vi "Distance.vi"(0 "X1":dbl, 1 "Y1":dbl, 2 "X2":dbl, 3 "Y2":dbl, 4 "X3":dbl, 5 "Y3":dbl, 6 "x4":dbl, 8 "Y":dbl, 9 "Y4":dbl, 10 "X":dbl) -> (14 "a2":dbl, 16 "a1":dbl, 17 "a3":dbl, 18 "Ra1":dbl, 19 "a4":dbl, 20 "A1":dbl, 21 "Ra2":dbl, 22 "Ra3":dbl, 23 "A2":dbl, 24 "Ra4":dbl, 25 "A3":dbl, 26 "A4":dbl)   [LabVIEW 2012]
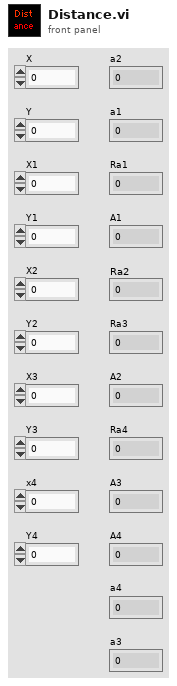
[diagram p1: front panel]
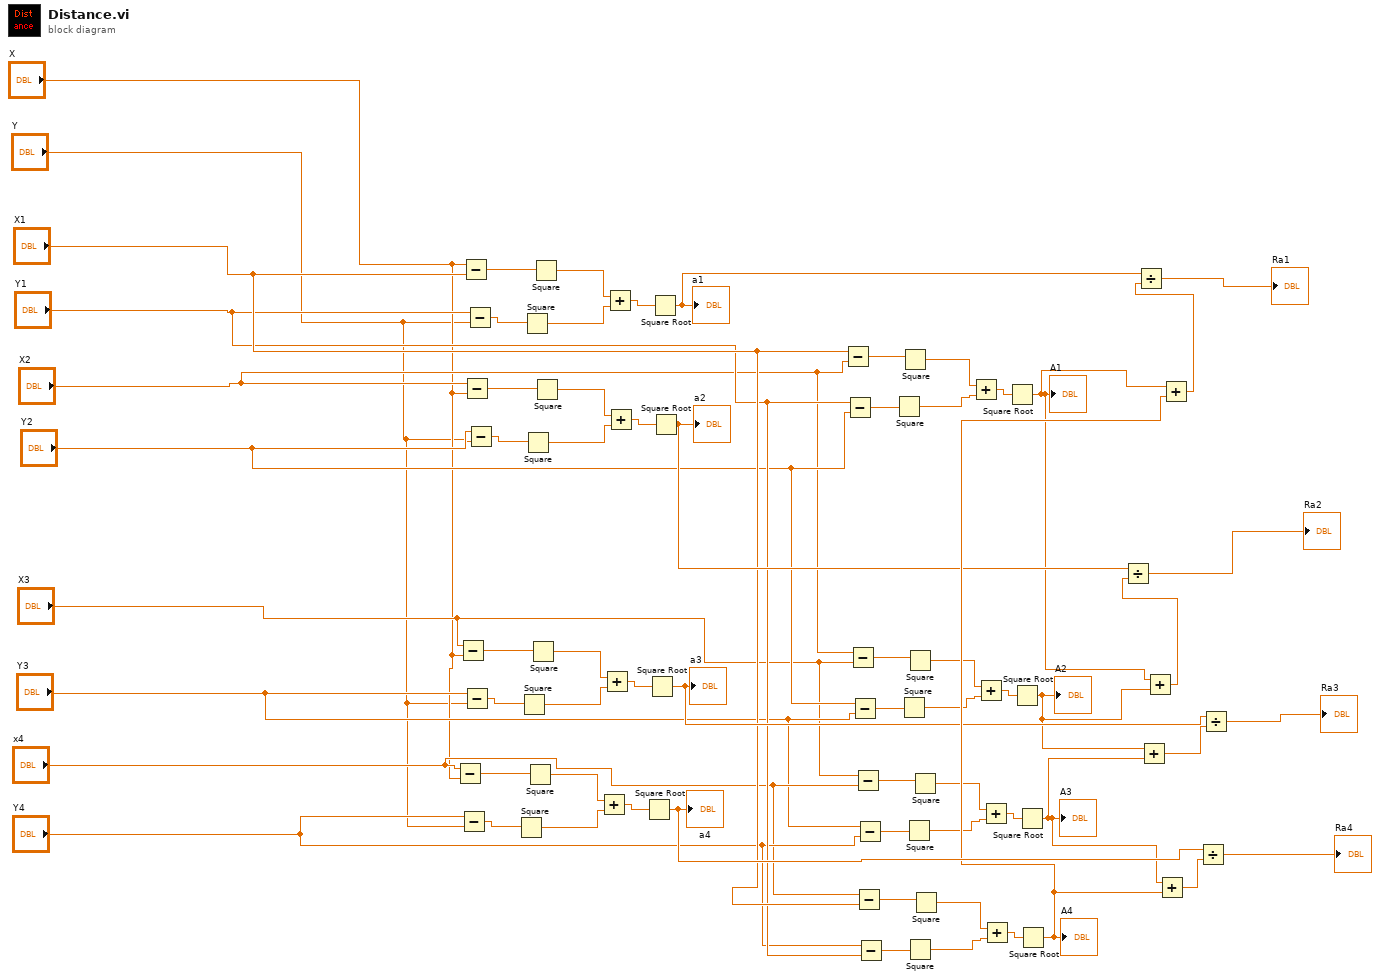
[diagram p0: block diagram]
diagram:
  n1 = Subtract(x="x4", y="X") -> (x-y=w17:dbl)
  n2 = Subtract(x="X3", y="X") -> (x-y=w12:dbl)
  n3 = Subtract(x="Y4", y="Y") -> (x-y=w18:dbl)
  n4 = Subtract(x="X", y="X1") -> (x-y=w2:dbl)
  n5 = Subtract(x="X2", y="X") -> (x-y=w7:dbl)
  n6 = Subtract(x="Y3", y="Y") -> (x-y=w13:dbl)
  n7 = Subtract(x="Y1", y="Y") -> (x-y=w3:dbl)
  n8 = Subtract(x="Y2", y="Y") -> (x-y=w8:dbl)
  n9 = Square(x=w18) -> (x^2=w20:dbl)
  n10 = Square(x=w13) -> (x^2=w15:dbl)
  n11 = Square(x=w3) -> (x^2=w5:dbl)
  n12 = Square(x=w8) -> (x^2=w10:dbl)
  n13 = Square(x=w17) -> (x^2=w19:dbl)
  n14 = Square(x=w12) -> (x^2=w14:dbl)
  n15 = Square(x=w2) -> (x^2=w4:dbl)
  n16 = Square(x=w7) -> (x^2=w9:dbl)
  n17 = Add(x=w19, y=w20) -> (x+y=w21:dbl)
  n18 = Add(x=w14, y=w15) -> (x+y=w16:dbl)
  n19 = Add(x=w4, y=w5) -> (x+y=w6:dbl)
  n20 = Add(x=w9, y=w10) -> (x+y=w11:dbl)
  n21 = Square Root(x=w21) -> (sqrt(x)=w65:dbl)
  "a4" <- w65
  n22 = Square Root(x=w16) -> (sqrt(x)=w59:dbl)
  "a3" <- w59
  n23 = Square Root(x=w6) -> (sqrt(x)=w52:dbl)
  "a1" <- w52
  n24 = Square Root(x=w11) -> (sqrt(x)=w56:dbl)
  "a2" <- w56
  n25 = Subtract(x="X1", y="X2") -> (x-y=w23:dbl)
  n26 = Subtract(x="Y1", y="Y2") -> (x-y=w24:dbl)
  n27 = Subtract(x="X2", y="X3") -> (x-y=w28:dbl)
  n28 = Subtract(x="Y2", y="Y3") -> (x-y=w29:dbl)
  n29 = Subtract(x="X3", y="x4") -> (x-y=w33:dbl)
  n30 = Subtract(x="x4", y="X1") -> (x-y=w40:dbl)
  n31 = Subtract(x="Y3", y="Y4") -> (x-y=w34:dbl)
  n32 = Subtract(x="Y4", y="Y1") -> (x-y=w41:dbl)
  n33 = Square(x=w24) -> (x^2=w26:dbl)
  n34 = Square(x=w29) -> (x^2=w31:dbl)
  n35 = Square(x=w23) -> (x^2=w25:dbl)
  n36 = Square(x=w34) -> (x^2=w36:dbl)
  n37 = Square(x=w28) -> (x^2=w30:dbl)
  n38 = Square(x=w41) -> (x^2=w43:dbl)
  n39 = Square(x=w33) -> (x^2=w35:dbl)
  n40 = Square(x=w40) -> (x^2=w42:dbl)
  n41 = Add(x=w25, y=w26) -> (x+y=w27:dbl)
  n42 = Add(x=w30, y=w31) -> (x+y=w32:dbl)
  n43 = Add(x=w35, y=w36) -> (x+y=w37:dbl)
  n44 = Add(x=w42, y=w43) -> (x+y=w44:dbl)
  n45 = Square Root(x=w27) -> (sqrt(x)=w54:dbl)
  "A1" <- w54
  n46 = Square Root(x=w32) -> (sqrt(x)=w58:dbl)
  "A2" <- w58
  n47 = Square Root(x=w37) -> (sqrt(x)=w62:dbl)
  "A3" <- w62
  n48 = Square Root(x=w44) -> (sqrt(x)=w63:dbl)
  "A4" <- w63
  n49 = Add(x=w58, y=w62) -> (x+y=w60:dbl)
  n50 = Add(x=w54, y=w58) -> (x+y=w55:dbl)
  n51 = Divide(x=w56, y=w55) -> (x/y=→"Ra2":dbl)
  n52 = Add(x=w62, y=w63) -> (x+y=w64:dbl)
  n53 = Add(x=w54, y=w63) -> (x+y=w51:dbl)
  n54 = Divide(x=w52, y=w51) -> (x/y=→"Ra1":dbl)
  n55 = Divide(x=w65, y=w64) -> (x/y=→"Ra4":dbl)
  n56 = Divide(x=w59, y=w60) -> (x/y=→"Ra3":dbl)
